vi "Main menu_4.vi"() -> ()   [LabVIEW 2022 SP3]
uses:
  <vilib>/event_ctls.llb/lveventtype.ctl
  <vilib>/Utility/file.llb/Write Delimited Spreadsheet (DBL).vi
panel:
  out "Close":bool
  in  "Close app":bool
  in  "?":T1(tab)
  in  "New plot":bool
  in  "Multicolumn Listbox":i32(listbox)
  in  "Close All plots":bool
  in  "CSV":bool
  in  "Start record":bool
  in  "Refresh \ntime (ms)":i32
  in  "Global Mode":enum32{"Item 0", "Item 1"}(radio)
  in  "Size bytes X #Traces":i32
  in  "Trace names":string(combo)
  in  "CTRL enable":bool
  in  "Save CTRL parameters":bool
  out "Total\ncontrols":i32
  in  "# Control":string(combo)
  in  "CS enable":bool
  out "Current CS status":i32
  in  "CS_IF_Params":T2 {"CS_Duty" min=0 max=1}
  out "Connected":bool
  out "Saved":bool
  in  "Save conf":bool
  in  "Port":i32
  in  "hostname":string
  in  "timeout ms":i32
  in  "Send message":bool
  in  "Process 2":i32
  in  "msj":string
  # "ctrl_if:0\nctrl: 2\nset parm: 2"
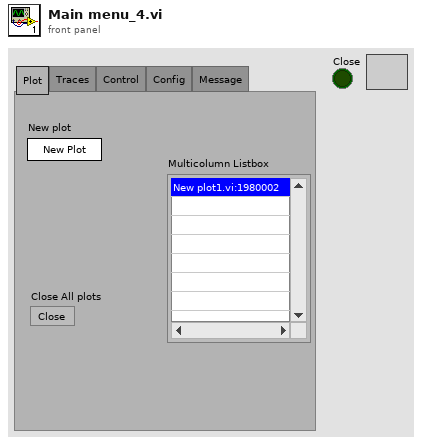
[diagram p1: front panel]
types:
  T1 = enum32{"Plot", "Traces", "Control", "Config", "Message"}
  T2 = cluster{"SET_PARAMETERS":i32, "CTLR":i32, "CS_Duty":sgl, "CTRL_IF_SET":i32}
  T3 = cluster{"Port":i32, "hostname":string, "status":bool, "timeout ms":i32, "TRACES_NAMES":string[], "Refresh time ms":i32, "Mode":enum32{"Item 0", "Item 1"}, "Start":bool, "DATA":sgl[][], "SIGNALS_NAMES":string[], "NB_SIGNALS":i32, "NB_TRACES":i32, "ID_TRACE":i32, "Mark":bool, "Counter":i32, "CTRLs_NAMES":string[], "NB_Ctrls":i32, "CS enable?":bool, "CS ID":i32}
  T4 = enum8{"Enabled", "Disabled", "Disabled and Grayed Out"}
  T5 = cluster{"TRACE_SIZE":i32, "CS_ID":i32, "TRACE ID":i32, "CMD":i32, "DATA PARAM":string}
  T6 = cluster{"TRACE_SIZE":i32, "CS_ID":i32, "TRACE ID":i32, "CMD":i32, "DATA(M)":i32}
  T7 = cluster{"timeout ms":i32, "remote port":u16, "Address":string}
  T8 = typedef "lveventtype.ctl" = enum32{"Null", "Timeout", "Annotation Menu Selection", "Annotation Menu Selection?", "App Instance Close", "App Instance Close?", "Autoscale Range Change", "Bookmark Info Change", "Cell Edit", "Cell Edit?", "Cursor Grab", "Cursor Grab?", "Cursor Menu Selection", "Cursor Menu Selection?", "Cursor Move", "Cursor Release", "Data Change", "Direction Change", "Display State Change", "Drag Ended", "Drag Enter", "Drag Leave", "Drag Over", "Drag Source Update", "Drag Starting", "Drag Starting?", "Drop", "Exec State Change", "Key Down", "Key Down?", "Key Repeat", "Key Repeat?", "Key Up", "Listbox Double Click", "Menu Activation?", "Menu Selection (App)", "Menu Selection? (App)", "Menu Selection (User)", "Mouse Down", "Mouse Down?", "Mouse Enter", "Mouse Leave", "Mouse Move", "Mouse Up", "Mouse Wheel", "NI Security User Change (App)", "Pane Size", "Panel Close", "Panel Close?", "Panel Resize", "Plot Attribute Change", "Scale Range Change", "Shortcut Menu Activation?", "Shortcut Menu Selection (App)", "Shortcut Menu Selection? (App)", "Shortcut Menu Selection (User)", "Tree Double Click", "Tree Drag", "Tree Drag?", "Tree Drop", "Tree Drop?", "Tree Item Close", "Tree Item Close?", "Tree Item Open", "Tree Item Open?", "User Event", "Value Change"}
  T9 = enum16{"open", "replace", "create", "open or create", "replace or create", "replace or create with confirmation"}
  T10 = enum16{"big-endian, network order", "native, host order", "little-endian"}
  T11 = cluster{"SIZE":i32, " TRACE DATA":sgl[], "TRACE_SIZE":i32, "NB_TRACES":i32, "NB_TRACED_SIGNALS":i32, "NAMES TRACED SIGNALS":string[], "NAMES TRACES":string[], "CS STATUS":i32, "NB_CSs":i32, "NAMES CSs":string[], "DATA (M)":sgl[], "CMD":i32}
  T12 = enum32{"invalid app kind", "Development System", "Run Time System", "Student Edition", "Embedded LabVIEW", "Evaluation", "Custom"}
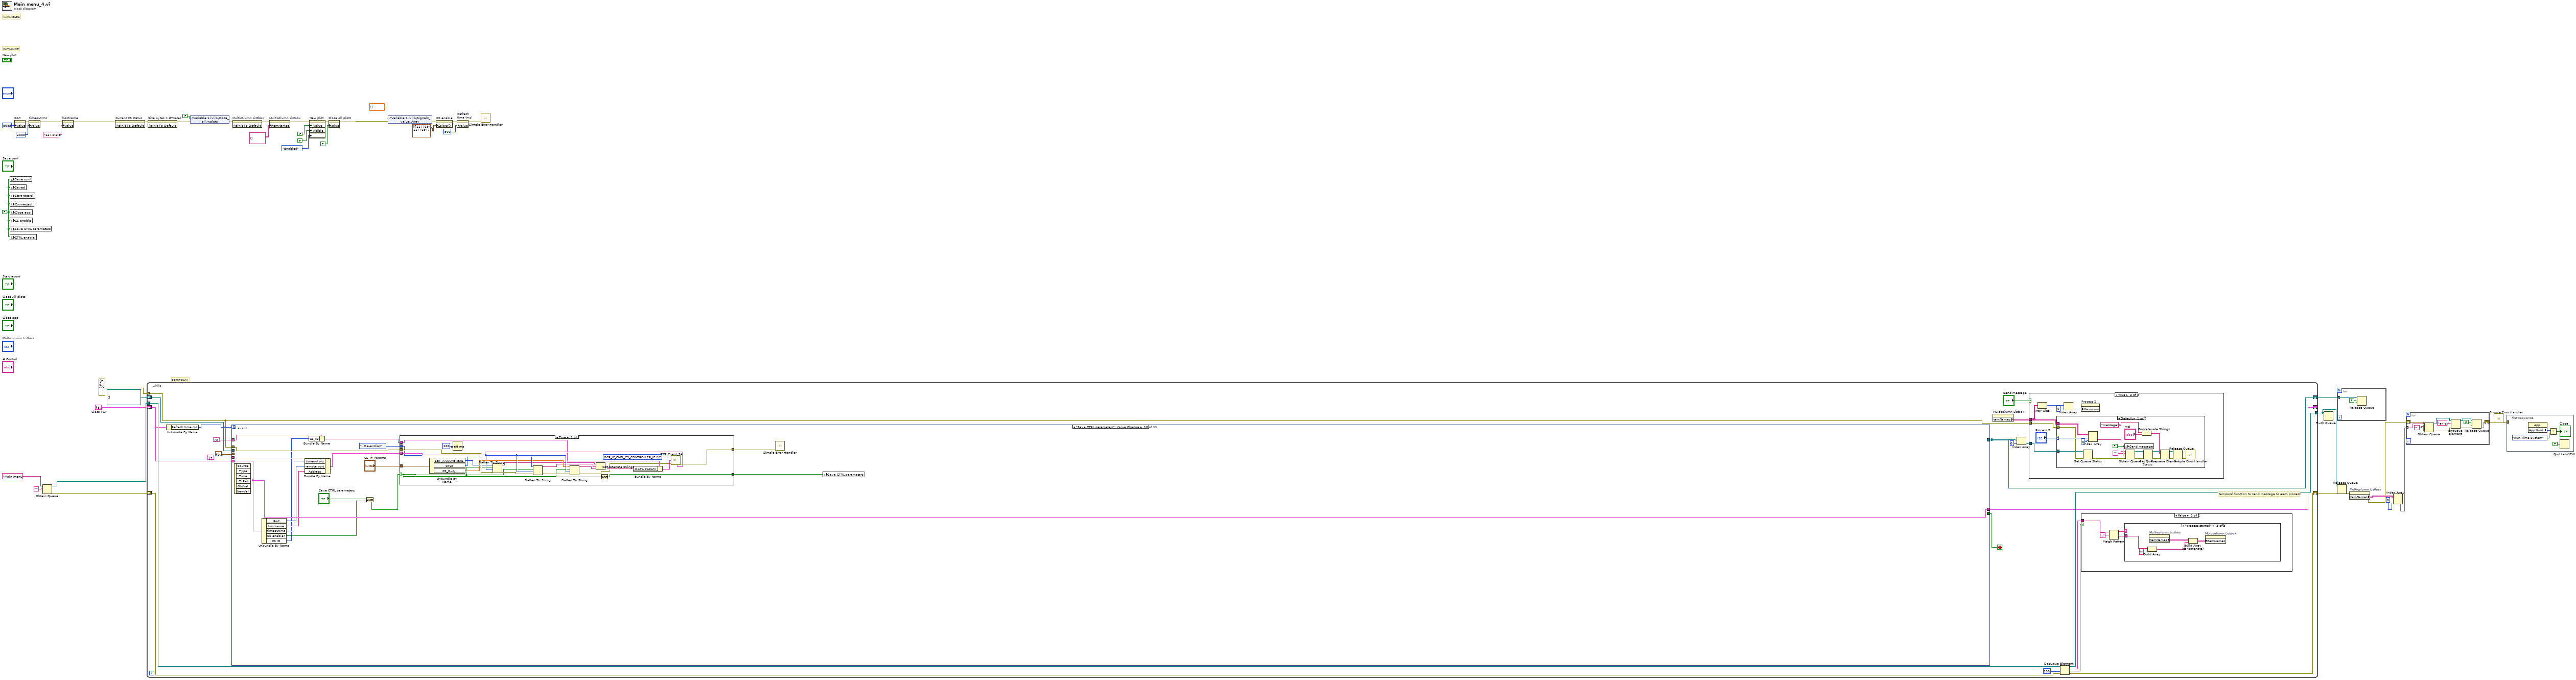
[diagram p0: block diagram]
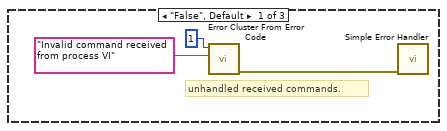
[diagram p4: hidden frame]
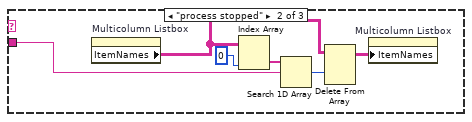
[diagram p5: hidden frame]
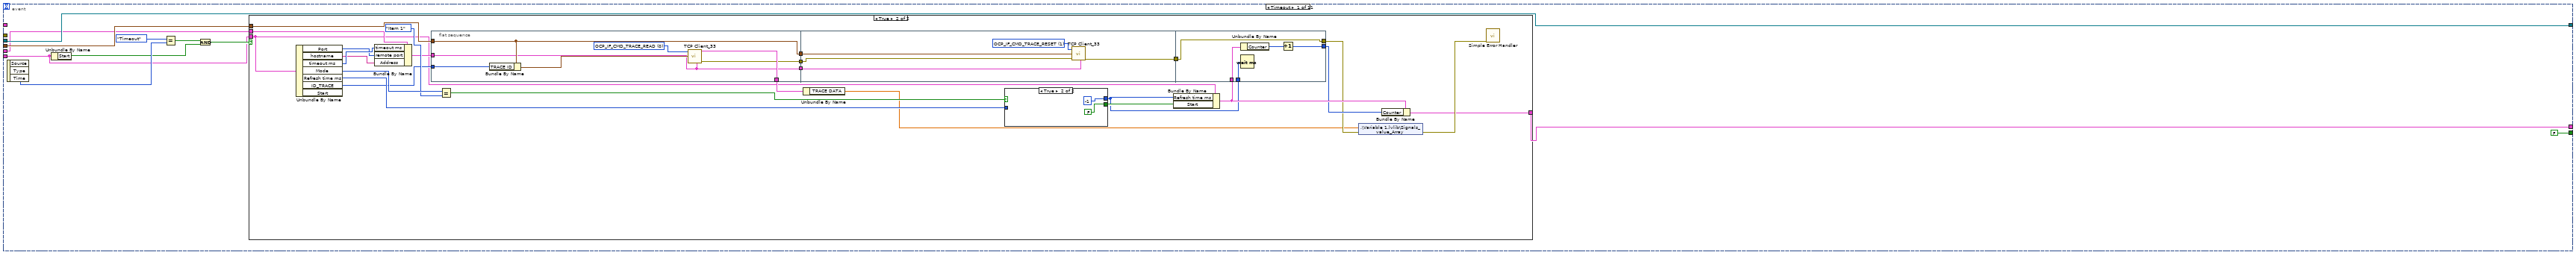
[diagram p7: hidden frame]
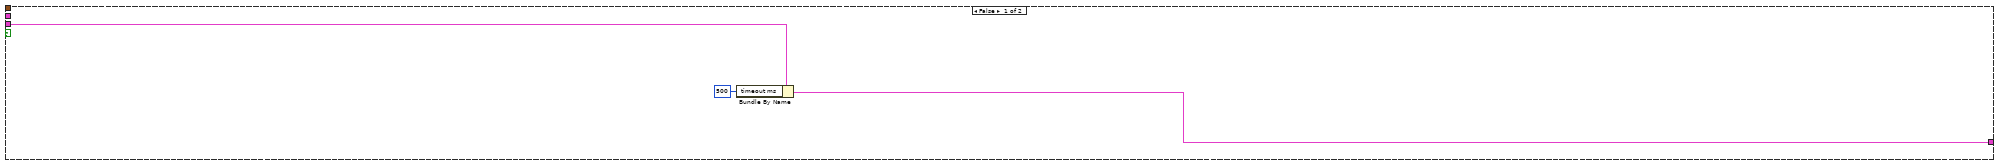
[diagram p8: hidden frame]
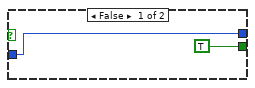
[diagram p9: hidden frame]
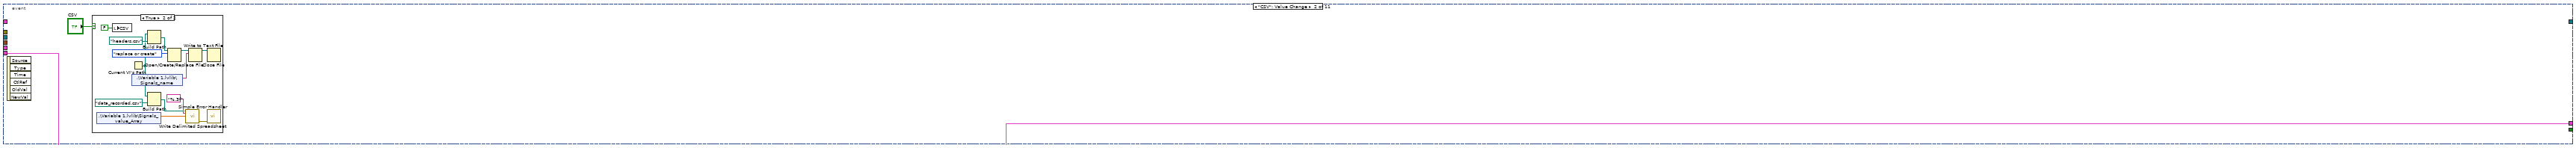
[diagram p10: hidden frame]
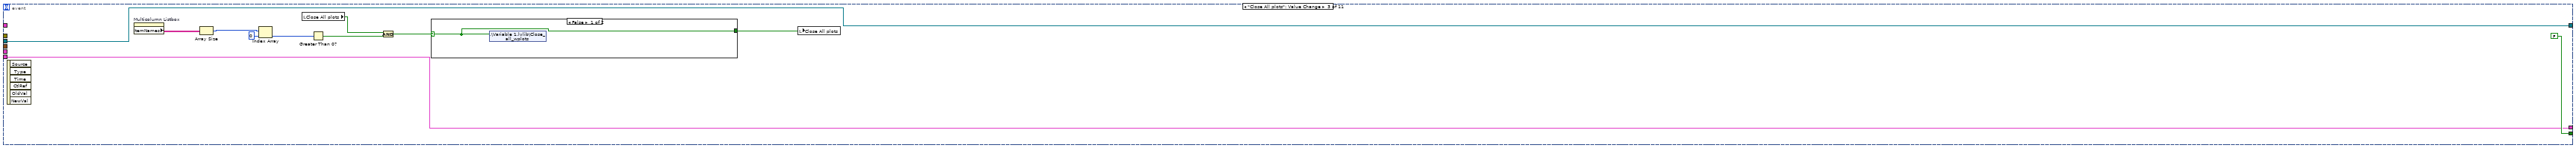
[diagram p12: hidden frame]
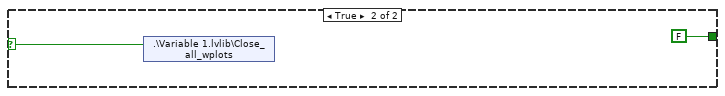
[diagram p13: hidden frame]
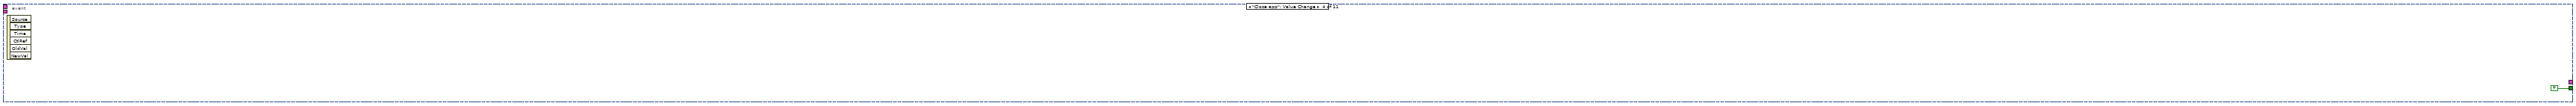
[diagram p14: hidden frame]
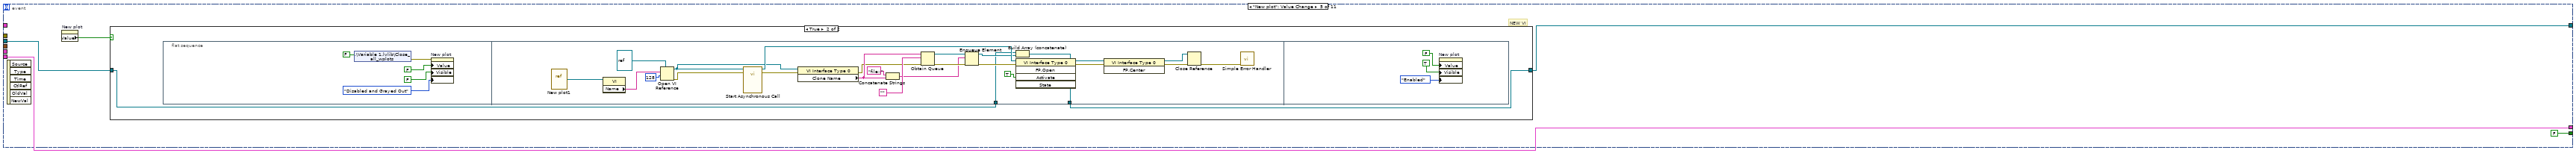
[diagram p15: hidden frame]
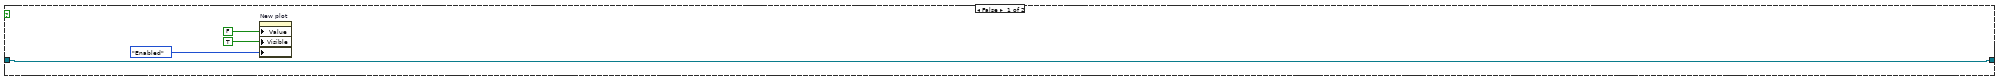
[diagram p16: hidden frame]
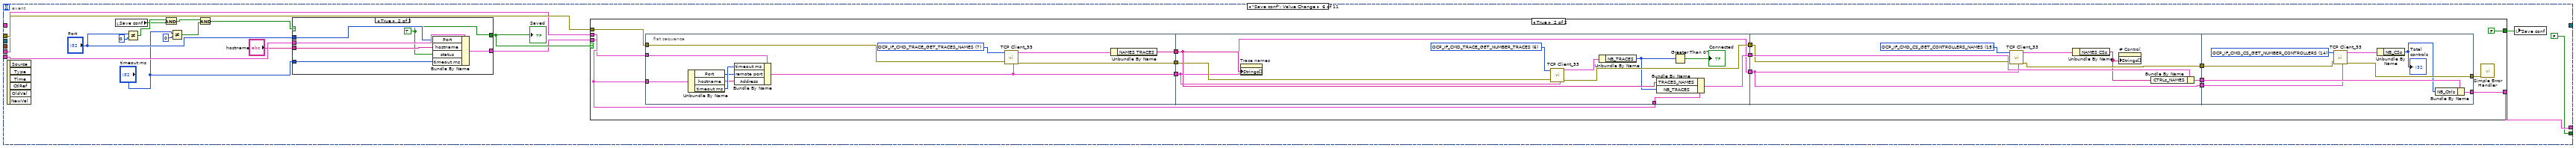
[diagram p17: hidden frame]
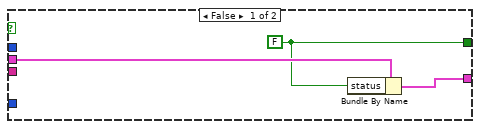
[diagram p19: hidden frame]
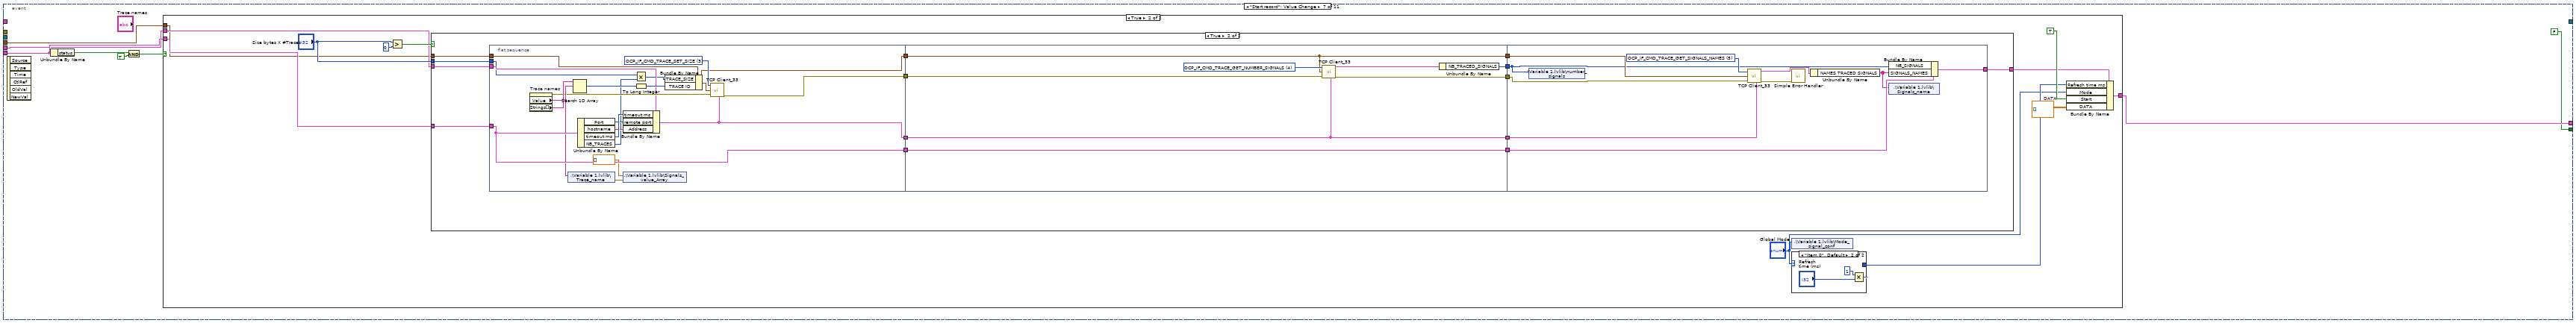
[diagram p20: hidden frame]
diagram:
  w22 = T3 {"Port"=8085, "hostname"="", "status"=FALSE, "timeout ms"=1000, "TRACES_NAMES"=[], "Refresh time ms"=500, "Mode"=enum."Item 0", "Start"=FALSE, "DATA"=[], "SIGNALS_NAMES"=[], "NB_SIGNALS"=0, "NB_TRACES"=0, "ID_TRACE"=0, "Mark"=FALSE, "Counter"=0, "CTRLs_NAMES"=[], "NB_Ctrls"=0, "CS enable?"=FALSE, "CS ID"=0}  # Class TCP
  w9 = FALSE ("Save conf")
  # "PROGRAM"
  # "INITIALIZE"
  # "VARIABLES"
  n1 = local write "Save conf"(w9) -> ()
  n2 = local write "Saved"(w9) -> ()
  n3 = local write "Start record"(w9) -> ()
  n4 = local write "Connected"(w9) -> ()
  n5 = local write "Close app"(w9) -> ()
  n6 = local write "CS enable"(w9) -> ()
  n7 = local write "Save CTRL parameters"(w9) -> ()
  n8 = local write "CTRL enable"(w9) -> ()
  n9 = property on="Port" class="DigNum (strict)"("Value"=8085) -> (error out=w20:errorcluster)  [unwired: 2 in, 1 out]
  n10 = property on="timeout ms" class="DigNum (strict)"(error in=w20, "Value"=2000 ("timeout ms")) -> (error out=w16:errorcluster)  [unwired: 1 in, 1 out]
  n11 = Obtain Queue(name (unnamed)="Main menu", element data type="") -> (queue out=w36:refnum<queue>, error out=w34:errorcluster)  [unwired: 3 in, 1 out]
  n12 = property on="hostname" class="Str"(error in=w16, "Value"="127.0.0.1" ("hostname")) -> (error out=w3:errorcluster)  [unwired: 1 in, 1 out]
  n13 = invoke on="Current CS status" class="DigNum (strict)" method="Reinit To Default"(error in=w3) -> (error out=w14:errorcluster)  [unwired: 2 in, 2 out]
  n14 = while {
    shift-right: [w48] -> w40
    shift-left: refnum<queue>[] [] -> [w63]
    tunnel: w36 -> [w62]
    tunnel: [w59] -> w26
    shift-right: [w53] -> w35
    shift-left: w34 -> [w58]
    shift-right: [w56] -> _
    shift-left: w22 -> [w55]
    tunnel: errorcluster {"status"=FALSE, "code"=0, "source"=""} ("error out") -> [w50]
    stop <- w64 stop-if-true
    # "temporal function to send message to each process"
    n15 = Unbundle By Name(w55) -> ("Refresh time ms"=w54:i32)
    n16 = event shown="[9] \"Save CTRL parameters\": Value Change" {
      selector: _ -> [_ _ _ _ _ _ _ _ _ _ _]
      dyn-events: _ -> [_ _ _ _ _ _ _ _ _ _ _]
      timeout: w54 -> [_ _ _ _ _ _ _ _ _ _ _]
      tunnel: [FALSE ("f") _ FALSE ("f") TRUE ("f") FALSE ("f") FALSE ("f") FALSE ("f") FALSE ("f") _ _ _] -> w64
      tunnel: [w119 _ w194 _ w202 _ _ _ _ _ _] -> w48
      tunnel: w63 -> [w119 _ w194 _ w201 _ _ _ _ _ _]
      tunnel: [w112 w169 w184 _ w199 w250 w328 w402 w445 w510 w561] -> w56
      tunnel: w55 -> [w113 w169 w184 _ w199 w258 w329 w402 w444 w510 w561]
      tunnel: w50 -> [_ _ _ _ _ w253 _ _ _ w511 w562]
      tunnel: T7 {"timeout ms"=2000, "remote port"=8085, "Address"="127.0.0.1"} ("Comunication Cluster") -> [w109 _ _ _ _ w243 w325 w406 w454 w507 w560]
      tunnel: T6 {"TRACE_SIZE"=0, "CS_ID"=0, "TRACE ID"=0, "CMD"=0, "DATA(M)"=0} ("Input Cluster") -> [w110 _ _ _ _ _ w324 w403 w453 _ _]
      tunnel: T5 {"TRACE_SIZE"=0, "CS_ID"=0, "TRACE ID"=0, "CMD"=0, "DATA PARAM"=""} ("Input Cluster") -> [_ _ _ _ _ _ _ _ _ w502 w555]
      event Timeout {
        n17 = event-data() -> ("Type"=w117:T8)  [unwired: 1 in, 2 out]
        n18 = Unbundle By Name(w113) -> ("Start"=w115:bool)
        n19 = Equal?(x=lveventtype."Timeout" ("Type"), y=w117) -> (x = y?=w116:bool)
        n20 = And(x=w116, y=w115) -> (x .and. y?=w114:bool)
        n21 = case shown="True" w114 {
          tunnel: w113 -> [w122 w123]
          tunnel: [w121 w137] -> w112
          tunnel: w110 -> [_ w126]
          tunnel: w109 -> [_ w125]
          frame False {
            n22 = Bundle By Name(cluster=w122, "timeout ms"=500) -> (w121:T3)
          }
          frame True {
            n23 = Unbundle By Name(w123) -> ("Port"=w131:i32, "hostname"=w130:string, "timeout ms"=w132:i32, "Mode"=w147:enum32{"Item 0", "Item 1"}, "Refresh time ms"=w144:i32, "ID_TRACE"=w141:i32)  [unwired: 1 out]
            n24 = Bundle By Name(cluster=w125, "timeout ms"=w132, "remote port"=w131, "Address"=w130) -> (w129:T7)
            n25 = flat-sequence {
              tunnel: w141 -> [w150]
              tunnel: [w154] -> w140
              tunnel: [w153] -> w139
              tunnel: w126 -> [w149]
              tunnel: [w149] -> w134
              tunnel: [w148] -> w133
              tunnel: w129 -> [w148]
              tunnel: w139 -> [w159]
              tunnel: w134 -> [w158]
              tunnel: w133 -> [w157]
              tunnel: [w155] -> w128
              tunnel: w138 -> [w164]
              tunnel: [w162] -> w136
              tunnel: w135 -> [w161]
              tunnel: w128 -> [w160]
              tunnel: [w160] -> w127
              frame #0 {
                w152 = 0 items=["OCP_IF_CMD_TRACE_READ", "OCP_IF_CMD_TRACE_RESET", "OCP_IF_CMD_TRACE_GET_SIZE", "OCP_IF_CMD_TRACE_SET_SIZE", "OCP_IF_CMD_TRACE_GET_NUMBER_SIGNALS", "OCP_IF_CMD_TRACE_GET_SIGNALS_NAMES", "OCP_IF_CMD_TRACE_GET_NUMBER_TRACES", "OCP_IF_CMD_TRACE_GET_TRACES_NAMES", "OCP_IF_CMD_TRACE_GET_ADDRESS", "OCP_IF_CMD_CS_STATUS", "OCP_IF_CMD_CS_ENABLE", "OCP_IF_CMD_CS_DISABLE", "OCP_IF_CMD_CS_CONTROLLER_IF", "OCP_IF_CMD_CS_HARDWARE_IF", "OCP_IF_CMD_CS_GET_NUMBER_CONTROLLERS", "OCP_IF_CMD_CS_GET_CONTROLLERS_NAMES", "OCP_IF_CMD_PLATFORM_ID", "OCP_IF_CMD_PLATFORM_IF", "OCP_IF_CMD_OPIL_UPDATE_MEASUREMENTS", "OCP_IF_CMD_OPIL_UPDATE_SIM_DATA", "OCP_IF_CMD_OPIL_RUN_CONTROL", "OCP_IF_CMD_OPIL_INITIALIZE_CONTROL", "OCP_IF_CMD_OPIL_GET_CONTROL", "OCP_IF_CMD_OPIL_GET_CONTROLLER_DATA", "OCP_IF_CMD_END"] ("CMD")
                n26 = Bundle By Name(cluster=w149, "TRACE ID"=w150) -> (w151:T6)
                n27 = call "TCP Client_33.vi"("CMD"=w152, "Input Cluster"=w151, "Comunication Cluster"=w148) -> ("Output cluster"=w154:T11, "error out"=w153:errorcluster)  [unwired: 5 in, 1 out]
              }
              frame #1 {
                w156 = 1 items=["OCP_IF_CMD_TRACE_READ", "OCP_IF_CMD_TRACE_RESET", "OCP_IF_CMD_TRACE_GET_SIZE", "OCP_IF_CMD_TRACE_SET_SIZE", "OCP_IF_CMD_TRACE_GET_NUMBER_SIGNALS", "OCP_IF_CMD_TRACE_GET_SIGNALS_NAMES", "OCP_IF_CMD_TRACE_GET_NUMBER_TRACES", "OCP_IF_CMD_TRACE_GET_TRACES_NAMES", "OCP_IF_CMD_TRACE_GET_ADDRESS", "OCP_IF_CMD_CS_STATUS", "OCP_IF_CMD_CS_ENABLE", "OCP_IF_CMD_CS_DISABLE", "OCP_IF_CMD_CS_CONTROLLER_IF", "OCP_IF_CMD_CS_HARDWARE_IF", "OCP_IF_CMD_CS_GET_NUMBER_CONTROLLERS", "OCP_IF_CMD_CS_GET_CONTROLLERS_NAMES", "OCP_IF_CMD_PLATFORM_ID", "OCP_IF_CMD_PLATFORM_IF", "OCP_IF_CMD_OPIL_UPDATE_MEASUREMENTS", "OCP_IF_CMD_OPIL_UPDATE_SIM_DATA", "OCP_IF_CMD_OPIL_RUN_CONTROL", "OCP_IF_CMD_OPIL_INITIALIZE_CONTROL", "OCP_IF_CMD_OPIL_GET_CONTROL", "OCP_IF_CMD_OPIL_GET_CONTROLLER_DATA", "OCP_IF_CMD_END"] ("CMD")
                n28 = call "TCP Client_33.vi"("CMD"=w156, "Input Cluster"=w158, "error in (no error)"=w159, "Comunication Cluster"=w157) -> ("error out"=w155:errorcluster)  [unwired: 4 in, 2 out]
              }
              frame #2 {
                n29 = Unbundle By Name(w164) -> ("Counter"=w163:i32)
                n30 = Wait (ms)(milliseconds to wait=w161) -> ()  [unwired: 1 out]
                n31 = Increment(x=w163) -> (x+1=w162:i32)
              }
            }
            n32 = Equal?(x=w147, y=enum32{"Item 0", "Item 1"}."Item 1" ("Mode")) -> (x = y?=w145:bool)
            n33 = Unbundle By Name(w140) -> ("TRACE DATA"=w124:sgl[])
            n34 = case shown="True" w145 {
              tunnel: [TRUE FALSE] -> w143
              tunnel: [w165 i8 -1 ("t")] -> w135
              tunnel: w144 -> [w165 _]
              frame False {
              }
              frame True {
              }
            }
            n35 = Bundle By Name(cluster=w123, "Refresh time ms"=w135, "Start"=w143) -> (w138:T3)
            n36 = shared-variable ".\\Variable 1.lvlib\\Signals_value_Array"(w124, error in=w127) -> (error out=w142:errorcluster)
            n37 = Bundle By Name(cluster=w138, "Counter"=w136) -> (w137:T3)
            n38 = call <vilib>:"Simple Error Handler.vi"("error in (no error)"=w142) -> ()  [unwired: 4 in, 5 out]
          }
        }
      }
      event "CSV": Value Change {
        n39 = event-data() -> ()  [unwired: 1 in, 6 out]
        n40 = case shown="True" "CSV" {
          frame False {
          }
          frame True {
            n41 = shared-variable ".\\Variable 1.lvlib\\Signals_value_Array"() -> (w180:dbl[])  [unwired: 1 in, 1 out]
            n42 = local write "CSV"(FALSE ("CSV")) -> ()
            n43 = Current VI's Path() -> (path=w171:path)
            n44 = shared-variable ".\\Variable 1.lvlib\\Signals_name"() -> (w174:string[])  [unwired: 1 in, 1 out]
            n45 = Build Path(base path=w171, name or relative path=path "headers.csv") -> (appended path=w177:path)
            n46 = Build Path(base path=w171, name or relative path=path "data_recorded.csv") -> (appended path=w179:path)
            n47 = Open/Create/Replace File(file path (use dialog)=w177, operation (0:open)=T9."replace or create") -> (refnum out=w175:refnum<file>)  [unwired: 4 in, 2 out]
            n48 = call-poly <vilib>:"Write Delimited Spreadsheet.vi"("file path (dialog if empty)"=w179, "format (%.3f)"="%.3f", "1D data"=w180) -> ("error out"=w181:errorcluster)  [unwired: 11 in, 1 out]
            n49 = Write to Text File(file (use dialog)=w175, text=w174) -> (refnum out=w173:refnum<file>)  [unwired: 2 in, 2 out]
            n50 = Close File(refnum=w173) -> ()  [unwired: 1 in, 2 out]
            n51 = call <vilib>:"Simple Error Handler.vi"("error in (no error)"=w181) -> ()  [unwired: 4 in, 5 out]
          }
        }
      }
      event "Close All plots": Value Change {
        n52 = event-data() -> ()  [unwired: 1 in, 6 out]
        n53 = property on="Multicolumn Listbox" class="MCListbox (strict)"() -> ("ItemNames"=w188:string[][])  [unwired: 2 in, 2 out]
        n54 = Array Size(array=w188) -> (size(s)=w192:i32[])
        n55 = Index Array(array=w192, index=0) -> (element=w190:i32)
        n56 = local read "Close All plots"() -> (w187:bool)
        n57 = Greater Than 0?(x=w190) -> (x > 0?=w185:bool)
        n58 = And(x=w187, y=w185) -> (x .and. y?=w186:bool)
        n59 = case shown="False" w186 {
          selector: w186 -> [w195 w196]
          tunnel: [w195 FALSE] -> w189
          frame False {
            n60 = shared-variable ".\\Variable 1.lvlib\\Close_all_wplots"(w195) -> ()  [unwired: 1 in, 1 out]
          }
          frame True {
            n61 = shared-variable ".\\Variable 1.lvlib\\Close_all_wplots"(w196) -> ()  [unwired: 1 in, 1 out]
          }
        }
        n62 = local write "Close All plots"(w189) -> ()
      }
      event "Close app": Value Change {
        n63 = event-data() -> ()  [unwired: 1 in, 6 out]
      }
      event "New plot": Value Change {
        # "NEW VI"
        n64 = event-data() -> ()  [unwired: 1 in, 6 out]
        n65 = property on="New plot" class="Bool (strict)"() -> ("Value"=w203:bool)  [unwired: 2 in, 2 out]
        n66 = case shown="True" w203 {
          tunnel: [w204 w209] -> w202
          tunnel: w201 -> [w204 w208]
          frame False {
            n67 = property on="New plot" class="Bool (strict)"("Value"=FALSE ("New plot"), "Visible"=TRUE, "DisabledEnum"=T4."Enabled" ("Disabled")) -> ()  [unwired: 2 in, 2 out]
          }
          frame True {
            n68 = flat-sequence {
              tunnel: [w220] -> w209
              tunnel: w208 -> [w219]
              frame #0 {
                n69 = shared-variable ".\\Variable 1.lvlib\\Close_all_wplots"(FALSE ("Close_all_wplots")) -> (error out=w210:errorcluster)  [unwired: 1 in]
                n70 = property on="New plot" class="Bool (strict)"(error in=w210, "Value"=FALSE ("New plot"), "Visible"=FALSE, "DisabledEnum"=T4."Disabled and Grayed Out" ("Disabled")) -> ()  [unwired: 1 in, 2 out]
              }
              frame #1 {
                n71 = vi-ref "New plot1.vi"() -> (w233:refnum<vi>)
                n72 = property class="VI"(reference=w233) -> ("Name"=w239:string)  [unwired: 1 in, 2 out]
                n73 = Open VI Reference(type specifier VI Refnum (for type only)=refnum<vi> refnum, vi path=w239, options=128) -> (vi reference=w230:refnum<vi>, error out=w235:errorcluster)  [unwired: 3 in]
                n74 = call-by-ref "Start Asynchronous Call"(reference=w230, error in=w235) -> (reference out=w234:refnum<vi>, error out=w224:errorcluster)  [unwired: 1 in, 1 out]
                n75 = property class="VI Interface Type 0"(reference=w230, error in=w224) -> (error out=w225:errorcluster, "Clone Name"=w227:string)  [unwired: 1 out]
                n76 = Concatenate Strings("file::" ("string"), w227) -> (w218:string)
                n77 = Obtain Queue(name (unnamed)=w227, element data type="", error in (no error)=w225) -> (queue out=w226:refnum<queue>, error out=w223:errorcluster)  [unwired: 2 in, 1 out]
                n78 = Enqueue Element(queue=w226, element=w218, error in (no error)=w223) -> (queue out=w221:refnum<queue>, error out=w222:errorcluster)  [unwired: 1 in, 1 out]
                n79 = Build Array (concatenate)(w219, w221) -> (w220:refnum<queue>[])
                n80 = invoke class="VI Interface Type 0" method="FP.Open"(reference=w234, error in=w222, "Activate"=TRUE ("Activate?")) -> (reference out=w232:refnum<vi>, error out=w217:errorcluster)  [unwired: 2 in, 3 out]
                n81 = invoke class="VI Interface Type 0" method="FP.Center"(reference=w232, error in=w217) -> (reference out=w231:refnum<vi>, error out=w216:errorcluster)  [unwired: 1 in, 1 out]
                n82 = Close Reference(reference=w231, error in (no error)=w216) -> (error out=w215:errorcluster)
                n83 = call <vilib>:"Simple Error Handler.vi"("error in (no error)"=w215) -> ()  [unwired: 4 in, 5 out]
              }
              frame #2 {
                n84 = property on="New plot" class="Bool (strict)"("Value"=FALSE ("Value (Signaling)"), "Visible"=TRUE, "DisabledEnum"=T4."Enabled" ("Disabled")) -> ()  [unwired: 2 in, 2 out]
              }
            }
          }
        }
      }
      event "Save conf": Value Change {
        n85 = event-data() -> ()  [unwired: 1 in, 6 out]
        n86 = local read "Save conf"() -> (w255:bool)
        n87 = Not Equal?(x="Port", y=0) -> (x != y?=w259:bool)
        n88 = And(x=w259, y=w255) -> (x .and. y?=w245:bool)
        n89 = Not Equal?(x="timeout ms", y=0) -> (x != y?=w247:bool)
        n90 = And(x=w245, y=w247) -> (x .and. y?=w246:bool)
        n91 = case shown="True" w246 {
          tunnel: [w315 w320] -> w254
          tunnel: "Port" -> [_ w322]
          tunnel: "hostname" -> [_ w321]
          tunnel: [w317 w318] -> w251
          tunnel: w258 -> [w316 w323]
          tunnel: "timeout ms" -> [_ w319]
          frame False {
            w315 = FALSE
            n92 = Bundle By Name(cluster=w316, "status"=w315) -> (w317:T3)
          }
          frame True {
            w320 = TRUE
            n93 = Bundle By Name(cluster=w323, "Port"=w322, "hostname"=w321, "status"=w320, "timeout ms"=w319) -> (w318:T3)
          }
        }
        "Saved" <- w254
        n94 = case shown="True" w254 {
          selector: w254 -> [w261 _]
          tunnel: w253 -> [_ w265]
          tunnel: [w261 FALSE] -> w252
          tunnel: w251 -> [w262 w276]
          tunnel: [w262 w275] -> w250
          tunnel: w243 -> [_ w263]
          frame False {
          }
          frame True {
            n95 = flat-sequence {
              tunnel: w276 -> [w288]
              tunnel: [w282] -> w274
              tunnel: [w281] -> w273
              tunnel: [w280] -> w272
              tunnel: w265 -> [w279]
              tunnel: w263 -> [w278]
              tunnel: w276 -> [w298]
              tunnel: w274 -> [w296]
              tunnel: w273 -> [w295]
              tunnel: w272 -> [w291]
              tunnel: [w297] -> w271
              tunnel: [w292] -> w269
              tunnel: [w291] -> w268
              tunnel: w271 -> [w306]
              tunnel: [w300] -> w270
              tunnel: w269 -> [w305]
              tunnel: w268 -> [w302]
              tunnel: [w303] -> w267
              tunnel: [w302] -> w266
              tunnel: [w310] -> w275
              tunnel: w270 -> [w314]
              tunnel: w267 -> [w313]
              tunnel: w266 -> [w312]
              tunnel: [w308] -> w264
              frame #0 {
                w287 = 7 items=["OCP_IF_CMD_TRACE_READ", "OCP_IF_CMD_TRACE_RESET", "OCP_IF_CMD_TRACE_GET_SIZE", "OCP_IF_CMD_TRACE_SET_SIZE", "OCP_IF_CMD_TRACE_GET_NUMBER_SIGNALS", "OCP_IF_CMD_TRACE_GET_SIGNALS_NAMES", "OCP_IF_CMD_TRACE_GET_NUMBER_TRACES", "OCP_IF_CMD_TRACE_GET_TRACES_NAMES", "OCP_IF_CMD_TRACE_GET_ADDRESS", "OCP_IF_CMD_CS_STATUS", "OCP_IF_CMD_CS_ENABLE", "OCP_IF_CMD_CS_DISABLE", "OCP_IF_CMD_CS_CONTROLLER_IF", "OCP_IF_CMD_CS_HARDWARE_IF", "OCP_IF_CMD_CS_GET_NUMBER_CONTROLLERS", "OCP_IF_CMD_CS_GET_CONTROLLERS_NAMES", "OCP_IF_CMD_PLATFORM_ID", "OCP_IF_CMD_PLATFORM_IF", "OCP_IF_CMD_OPIL_UPDATE_MEASUREMENTS", "OCP_IF_CMD_OPIL_UPDATE_SIM_DATA", "OCP_IF_CMD_OPIL_RUN_CONTROL", "OCP_IF_CMD_OPIL_INITIALIZE_CONTROL", "OCP_IF_CMD_OPIL_GET_CONTROL", "OCP_IF_CMD_OPIL_GET_CONTROLLER_DATA", "OCP_IF_CMD_END"] ("CMD")
                n96 = Unbundle By Name(w288) -> ("Port"=w284:i32, "hostname"=w283:string, "timeout ms"=w285:i32)
                n97 = Bundle By Name(cluster=w278, "timeout ms"=w285, "remote port"=w284, "Address"=w283) -> (w280:T7)
                n98 = call "TCP Client_33.vi"("CMD"=w287, "error in (no error)"=w279, "Comunication Cluster"=w280) -> ("Output cluster"=w286:T11, "error out"=w281:errorcluster)  [unwired: 5 in, 1 out]
                n99 = Unbundle By Name(w286) -> ("NAMES TRACES"=w282:string[])
              }
              frame #1 {
                w294 = 6 items=["OCP_IF_CMD_TRACE_READ", "OCP_IF_CMD_TRACE_RESET", "OCP_IF_CMD_TRACE_GET_SIZE", "OCP_IF_CMD_TRACE_SET_SIZE", "OCP_IF_CMD_TRACE_GET_NUMBER_SIGNALS", "OCP_IF_CMD_TRACE_GET_SIGNALS_NAMES", "OCP_IF_CMD_TRACE_GET_NUMBER_TRACES", "OCP_IF_CMD_TRACE_GET_TRACES_NAMES", "OCP_IF_CMD_TRACE_GET_ADDRESS", "OCP_IF_CMD_CS_STATUS", "OCP_IF_CMD_CS_ENABLE", "OCP_IF_CMD_CS_DISABLE", "OCP_IF_CMD_CS_CONTROLLER_IF", "OCP_IF_CMD_CS_HARDWARE_IF", "OCP_IF_CMD_CS_GET_NUMBER_CONTROLLERS", "OCP_IF_CMD_CS_GET_CONTROLLERS_NAMES", "OCP_IF_CMD_PLATFORM_ID", "OCP_IF_CMD_PLATFORM_IF", "OCP_IF_CMD_OPIL_UPDATE_MEASUREMENTS", "OCP_IF_CMD_OPIL_UPDATE_SIM_DATA", "OCP_IF_CMD_OPIL_RUN_CONTROL", "OCP_IF_CMD_OPIL_INITIALIZE_CONTROL", "OCP_IF_CMD_OPIL_GET_CONTROL", "OCP_IF_CMD_OPIL_GET_CONTROLLER_DATA", "OCP_IF_CMD_END"] ("CMD")
                n100 = property on="Trace names" class="CmbBox"("Strings[]"=w296) -> ()  [unwired: 2 in, 2 out]
                n101 = call "TCP Client_33.vi"("CMD"=w294, "error in (no error)"=w295, "Comunication Cluster"=w291) -> ("Output cluster"=w293:T11, "error out"=w292:errorcluster)  [unwired: 5 in, 1 out]
                n102 = Unbundle By Name(w293) -> ("NB_TRACES"=w290:i32)
                n103 = Bundle By Name(cluster=w298, "TRACES_NAMES"=w296, "NB_TRACES"=w290) -> (w297:T3)
                n104 = Greater Than 0?(x=w290) -> (x > 0?=→"Connected":bool)
              }
              frame #2 {
                w304 = 15 items=["OCP_IF_CMD_TRACE_READ", "OCP_IF_CMD_TRACE_RESET", "OCP_IF_CMD_TRACE_GET_SIZE", "OCP_IF_CMD_TRACE_SET_SIZE", "OCP_IF_CMD_TRACE_GET_NUMBER_SIGNALS", "OCP_IF_CMD_TRACE_GET_SIGNALS_NAMES", "OCP_IF_CMD_TRACE_GET_NUMBER_TRACES", "OCP_IF_CMD_TRACE_GET_TRACES_NAMES", "OCP_IF_CMD_TRACE_GET_ADDRESS", "OCP_IF_CMD_CS_STATUS", "OCP_IF_CMD_CS_ENABLE", "OCP_IF_CMD_CS_DISABLE", "OCP_IF_CMD_CS_CONTROLLER_IF", "OCP_IF_CMD_CS_HARDWARE_IF", "OCP_IF_CMD_CS_GET_NUMBER_CONTROLLERS", "OCP_IF_CMD_CS_GET_CONTROLLERS_NAMES", "OCP_IF_CMD_PLATFORM_ID", "OCP_IF_CMD_PLATFORM_IF", "OCP_IF_CMD_OPIL_UPDATE_MEASUREMENTS", "OCP_IF_CMD_OPIL_UPDATE_SIM_DATA", "OCP_IF_CMD_OPIL_RUN_CONTROL", "OCP_IF_CMD_OPIL_INITIALIZE_CONTROL", "OCP_IF_CMD_OPIL_GET_CONTROL", "OCP_IF_CMD_OPIL_GET_CONTROLLER_DATA", "OCP_IF_CMD_END"] ("CMD")
                n105 = call "TCP Client_33.vi"("CMD"=w304, "error in (no error)"=w305, "Comunication Cluster"=w302) -> ("Output cluster"=w301:T11, "error out"=w303:errorcluster)  [unwired: 5 in, 1 out]
                n106 = Unbundle By Name(w301) -> ("NAMES CSs"=w299:string[])
                n107 = property on="# Control" class="CmbBox"("Strings[]"=w299) -> ()  [unwired: 2 in, 2 out]
                n108 = Bundle By Name(cluster=w306, "CTRLs_NAMES"=w299) -> (w300:T3)
              }
              frame #3 {
                w311 = 14 items=["OCP_IF_CMD_TRACE_READ", "OCP_IF_CMD_TRACE_RESET", "OCP_IF_CMD_TRACE_GET_SIZE", "OCP_IF_CMD_TRACE_SET_SIZE", "OCP_IF_CMD_TRACE_GET_NUMBER_SIGNALS", "OCP_IF_CMD_TRACE_GET_SIGNALS_NAMES", "OCP_IF_CMD_TRACE_GET_NUMBER_TRACES", "OCP_IF_CMD_TRACE_GET_TRACES_NAMES", "OCP_IF_CMD_TRACE_GET_ADDRESS", "OCP_IF_CMD_CS_STATUS", "OCP_IF_CMD_CS_ENABLE", "OCP_IF_CMD_CS_DISABLE", "OCP_IF_CMD_CS_CONTROLLER_IF", "OCP_IF_CMD_CS_HARDWARE_IF", "OCP_IF_CMD_CS_GET_NUMBER_CONTROLLERS", "OCP_IF_CMD_CS_GET_CONTROLLERS_NAMES", "OCP_IF_CMD_PLATFORM_ID", "OCP_IF_CMD_PLATFORM_IF", "OCP_IF_CMD_OPIL_UPDATE_MEASUREMENTS", "OCP_IF_CMD_OPIL_UPDATE_SIM_DATA", "OCP_IF_CMD_OPIL_RUN_CONTROL", "OCP_IF_CMD_OPIL_INITIALIZE_CONTROL", "OCP_IF_CMD_OPIL_GET_CONTROL", "OCP_IF_CMD_OPIL_GET_CONTROLLER_DATA", "OCP_IF_CMD_END"] ("CMD")
                n109 = call "TCP Client_33.vi"("CMD"=w311, "error in (no error)"=w313, "Comunication Cluster"=w312) -> ("Output cluster"=w309:T11, "error out"=w308:errorcluster)  [unwired: 5 in, 1 out]
                n110 = Unbundle By Name(w309) -> ("NB_CSs"=w307:i32)
                "Total\ncontrols" <- w307
                n111 = Bundle By Name(cluster=w314, "NB_Ctrls"=w307) -> (w310:T3)
              }
            }
            n112 = call <vilib>:"Simple Error Handler.vi"("error in (no error)"=w264) -> ()  [unwired: 4 in, 5 out]
          }
        }
        n113 = local write "Save conf"(w252) -> ()
      }
      event "Start record": Value Change {
        n114 = event-data() -> ()  [unwired: 1 in, 6 out]
        n115 = Unbundle By Name(w329) -> ("status"=w331:bool)
        n116 = And(x=w331, y=TRUE) -> (x .and. y?=w330:bool)
        n117 = case shown="True" w330 {
          tunnel: w329 -> [w332 w338]
          tunnel: [w332 w344] -> w328
          tunnel: w325 -> [_ w335]
          tunnel: w324 -> [_ w334]
          frame False {
          }
          frame True {
            w333 = sgl[][] []  # DATA
            n118 = Greater?(x="Size bytes X #Traces", y=0) -> (0:w340:bool)
            n119 = case shown="True" w340 {
              tunnel: "Size bytes X #Traces" -> [_ w359]
              tunnel: w338 -> [w345 w358]
              tunnel: [w345 w354] -> w337
              tunnel: w335 -> [_ w347]
              tunnel: w334 -> [_ w346]
              frame False {
              }
              frame True {
                n120 = flat-sequence {
                  tunnel: w359 -> [w363]
                  tunnel: w358 -> [w379]
                  tunnel: [w375] -> w357
                  tunnel: [w379] -> w356
                  tunnel: [w368] -> w353
                  tunnel: [w367] -> w352
                  tunnel: w347 -> [w366]
                  tunnel: w346 -> [w365]
                  tunnel: w357 -> [w386]
                  tunnel: w356 -> [w387]
                  tunnel: [w387] -> w355
                  tunnel: w353 -> [w380]
                  tunnel: w352 -> [w381]
                  tunnel: [w383] -> w351
                  tunnel: [w382] -> w350
                  tunnel: [w381] -> w349
                  tunnel: [w380] -> w348
                  tunnel: w355 -> [w397]
                  tunnel: [w396] -> w354
                  tunnel: w351 -> [w388]
                  tunnel: w350 -> [w392]
                  tunnel: w349 -> [w390]
                  tunnel: w348 -> [w389]
                  frame #0 {
                    w374 = 3 items=["OCP_IF_CMD_TRACE_READ", "OCP_IF_CMD_TRACE_RESET", "OCP_IF_CMD_TRACE_GET_SIZE", "OCP_IF_CMD_TRACE_SET_SIZE", "OCP_IF_CMD_TRACE_GET_NUMBER_SIGNALS", "OCP_IF_CMD_TRACE_GET_SIGNALS_NAMES", "OCP_IF_CMD_TRACE_GET_NUMBER_TRACES", "OCP_IF_CMD_TRACE_GET_TRACES_NAMES", "OCP_IF_CMD_TRACE_GET_ADDRESS", "OCP_IF_CMD_CS_STATUS", "OCP_IF_CMD_CS_ENABLE", "OCP_IF_CMD_CS_DISABLE", "OCP_IF_CMD_CS_CONTROLLER_IF", "OCP_IF_CMD_CS_HARDWARE_IF", "OCP_IF_CMD_CS_GET_NUMBER_CONTROLLERS", "OCP_IF_CMD_CS_GET_CONTROLLERS_NAMES", "OCP_IF_CMD_PLATFORM_ID", "OCP_IF_CMD_PLATFORM_IF", "OCP_IF_CMD_OPIL_UPDATE_MEASUREMENTS", "OCP_IF_CMD_OPIL_UPDATE_SIM_DATA", "OCP_IF_CMD_OPIL_RUN_CONTROL", "OCP_IF_CMD_OPIL_INITIALIZE_CONTROL", "OCP_IF_CMD_OPIL_GET_CONTROL", "OCP_IF_CMD_OPIL_GET_CONTROLLER_DATA", "OCP_IF_CMD_END"] ("CMD")
                    n121 = property on="Trace names" class="CmbBox"() -> (error out=w370:errorcluster, "Value"=w376:string, "Strings[]"=w378:string[])  [unwired: 2 in, 1 out]
                    n122 = shared-variable ".\\Variable 1.lvlib\\Trace_name"(w376) -> (error out=w361:errorcluster)  [unwired: 1 in]
                    n123 = Search 1D Array(1D array=w378, element=w376) -> (index of element=w377:i32)  [unwired: 1 in]
                    n124 = Unbundle By Name(w379) -> ("Port"=w372:i32, "hostname"=w371:string, "timeout ms"=w373:i32, "NB_TRACES"=w364:i32)
                    n125 = Bundle By Name(cluster=w366, "timeout ms"=w373, "remote port"=w372, "Address"=w371) -> (w367:T7)
                    n126 = shared-variable ".\\Variable 1.lvlib\\Signals_value_Array"(dbl[] [] ("Signals_value_Array"), error in=w361) -> ()  [unwired: 1 out]
                    n127 = Multiply(x=w363, y=w364) -> (x*y=w362:i32)
                    n128 = To Long Integer(number=w377) -> (32bit integer=w369:i32)
                    n129 = Bundle By Name(cluster=w365, "TRACE_SIZE"=w362, "TRACE ID"=w369) -> (w368:T6)
                    n130 = call "TCP Client_33.vi"("CMD"=w374, "Input Cluster"=w368, "error in (no error)"=w370, "Comunication Cluster"=w367) -> ("error out"=w375:errorcluster)  [unwired: 4 in, 2 out]
                  }
                  frame #1 {
                    w385 = 4 items=["OCP_IF_CMD_TRACE_READ", "OCP_IF_CMD_TRACE_RESET", "OCP_IF_CMD_TRACE_GET_SIZE", "OCP_IF_CMD_TRACE_SET_SIZE", "OCP_IF_CMD_TRACE_GET_NUMBER_SIGNALS", "OCP_IF_CMD_TRACE_GET_SIGNALS_NAMES", "OCP_IF_CMD_TRACE_GET_NUMBER_TRACES", "OCP_IF_CMD_TRACE_GET_TRACES_NAMES", "OCP_IF_CMD_TRACE_GET_ADDRESS", "OCP_IF_CMD_CS_STATUS", "OCP_IF_CMD_CS_ENABLE", "OCP_IF_CMD_CS_DISABLE", "OCP_IF_CMD_CS_CONTROLLER_IF", "OCP_IF_CMD_CS_HARDWARE_IF", "OCP_IF_CMD_CS_GET_NUMBER_CONTROLLERS", "OCP_IF_CMD_CS_GET_CONTROLLERS_NAMES", "OCP_IF_CMD_PLATFORM_ID", "OCP_IF_CMD_PLATFORM_IF", "OCP_IF_CMD_OPIL_UPDATE_MEASUREMENTS", "OCP_IF_CMD_OPIL_UPDATE_SIM_DATA", "OCP_IF_CMD_OPIL_RUN_CONTROL", "OCP_IF_CMD_OPIL_INITIALIZE_CONTROL", "OCP_IF_CMD_OPIL_GET_CONTROL", "OCP_IF_CMD_OPIL_GET_CONTROLLER_DATA", "OCP_IF_CMD_END"] ("CMD")
                    n131 = call "TCP Client_33.vi"("CMD"=w385, "Input Cluster"=w380, "error in (no error)"=w386, "Comunication Cluster"=w381) -> ("Output cluster"=w384:T11, "error out"=w382:errorcluster)  [unwired: 4 in, 1 out]
                    n132 = Unbundle By Name(w384) -> ("NB_TRACED_SIGNALS"=w383:i32)
                  }
                  frame #2 {
                    w391 = 5 items=["OCP_IF_CMD_TRACE_READ", "OCP_IF_CMD_TRACE_RESET", "OCP_IF_CMD_TRACE_GET_SIZE", "OCP_IF_CMD_TRACE_SET_SIZE", "OCP_IF_CMD_TRACE_GET_NUMBER_SIGNALS", "OCP_IF_CMD_TRACE_GET_SIGNALS_NAMES", "OCP_IF_CMD_TRACE_GET_NUMBER_TRACES", "OCP_IF_CMD_TRACE_GET_TRACES_NAMES", "OCP_IF_CMD_TRACE_GET_ADDRESS", "OCP_IF_CMD_CS_STATUS", "OCP_IF_CMD_CS_ENABLE", "OCP_IF_CMD_CS_DISABLE", "OCP_IF_CMD_CS_CONTROLLER_IF", "OCP_IF_CMD_CS_HARDWARE_IF", "OCP_IF_CMD_CS_GET_NUMBER_CONTROLLERS", "OCP_IF_CMD_CS_GET_CONTROLLERS_NAMES", "OCP_IF_CMD_PLATFORM_ID", "OCP_IF_CMD_PLATFORM_IF", "OCP_IF_CMD_OPIL_UPDATE_MEASUREMENTS", "OCP_IF_CMD_OPIL_UPDATE_SIM_DATA", "OCP_IF_CMD_OPIL_RUN_CONTROL", "OCP_IF_CMD_OPIL_INITIALIZE_CONTROL", "OCP_IF_CMD_OPIL_GET_CONTROL", "OCP_IF_CMD_OPIL_GET_CONTROLLER_DATA", "OCP_IF_CMD_END"] ("CMD")
                    n133 = shared-variable ".\\Variable 1.lvlib\\number_signals"(w388) -> ()  [unwired: 1 in, 1 out]
                    n134 = call "TCP Client_33.vi"("CMD"=w391, "Input Cluster"=w389, "error in (no error)"=w392, "Comunication Cluster"=w390) -> ("Output cluster"=w395:T11, "error out"=w393:errorcluster)  [unwired: 4 in, 1 out]
                    n135 = call <vilib>:"Simple Error Handler.vi"("error in (no error)"=w393) -> ()  [unwired: 4 in, 5 out]
                    n136 = Unbundle By Name(w395) -> ("NAMES TRACED SIGNALS"=w394:string[])
                    n137 = Bundle By Name(cluster=w397, "NB_SIGNALS"=w388, "SIGNALS_NAMES"=w394) -> (w396:T3)
                    n138 = shared-variable ".\\Variable 1.lvlib\\Signals_name"(w394) -> ()  [unwired: 1 in, 1 out]
                  }
                }
              }
            }
            n139 = shared-variable ".\\Variable 1.lvlib\\Mode_signal_conf"("Global Mode") -> ()  [unwired: 1 in, 1 out]
            n140 = case shown="\"Item 0\", Default" "Global Mode" {
              tunnel: [200 ("Refresh time (sec)") w399] -> w342
              frame "Item 1" {
              }
              frame "Item 0", Default {
                n141 = Multiply(x=1, y="Refresh \ntime (ms)") -> (x*y=w399:i32)
              }
            }
            n142 = Bundle By Name(cluster=w337, "Refresh time ms"=w342, "Mode"="Global Mode", "Start"=TRUE, "DATA"=w333) -> (w344:T3)
          }
        }
      }
      event "Trace names", "# Control": Value Change {
        n143 = event-data() -> ()  [unwired: 1 in, 6 out]
        n144 = Unbundle By Name(w402) -> ("Port"=w410:i32, "hostname"=w409:string, "timeout ms"=w408:i32)
        n145 = Bundle By Name(cluster=w406, "timeout ms"=w408, "remote port"=w410, "Address"=w409) -> (w405:T7)
        n146 = flat-sequence {
          tunnel: w403 -> [w424]
          tunnel: [w424] -> w411
          tunnel: [w426] -> w407
          tunnel: w405 -> [w425]
          tunnel: [w425] -> w404
          tunnel: [w437] -> w412
          tunnel: w411 -> [w441]
          tunnel: w407 -> [w436]
          tunnel: w404 -> [w435]
          frame #0 {
            w427 = 2 items=["OCP_IF_CMD_TRACE_READ", "OCP_IF_CMD_TRACE_RESET", "OCP_IF_CMD_TRACE_GET_SIZE", "OCP_IF_CMD_TRACE_SET_SIZE", "OCP_IF_CMD_TRACE_GET_NUMBER_SIGNALS", "OCP_IF_CMD_TRACE_GET_SIGNALS_NAMES", "OCP_IF_CMD_TRACE_GET_NUMBER_TRACES", "OCP_IF_CMD_TRACE_GET_TRACES_NAMES", "OCP_IF_CMD_TRACE_GET_ADDRESS", "OCP_IF_CMD_CS_STATUS", "OCP_IF_CMD_CS_ENABLE", "OCP_IF_CMD_CS_DISABLE", "OCP_IF_CMD_CS_CONTROLLER_IF", "OCP_IF_CMD_CS_HARDWARE_IF", "OCP_IF_CMD_CS_GET_NUMBER_CONTROLLERS", "OCP_IF_CMD_CS_GET_CONTROLLERS_NAMES", "OCP_IF_CMD_PLATFORM_ID", "OCP_IF_CMD_PLATFORM_IF", "OCP_IF_CMD_OPIL_UPDATE_MEASUREMENTS", "OCP_IF_CMD_OPIL_UPDATE_SIM_DATA", "OCP_IF_CMD_OPIL_RUN_CONTROL", "OCP_IF_CMD_OPIL_INITIALIZE_CONTROL", "OCP_IF_CMD_OPIL_GET_CONTROL", "OCP_IF_CMD_OPIL_GET_CONTROLLER_DATA", "OCP_IF_CMD_END"] ("CMD")
            n147 = property on="Trace names" class="CmbBox"() -> ("Value"=w419:string, "Strings[]"=w420:string[])  [unwired: 2 in, 2 out]
            n148 = Search 1D Array(1D array=w420, element=w419) -> (index of element=w415:i32)  [unwired: 1 in]
            n149 = Less Than 0?(x=w415) -> (x < 0?=w416:bool)
            n150 = Select(t=0, s=w416, f=w415) -> (s? t:f=w414:i32)
            n151 = To Long Integer(number=w414) -> (32bit integer=w418:i32)
            n152 = Bundle By Name(cluster=w424, "TRACE ID"=w418) -> (w423:T6)
            n153 = call "TCP Client_33.vi"("CMD"=w427, "Input Cluster"=w423, "Comunication Cluster"=w425) -> ("Output cluster"=w421:T11, "error out"=w426:errorcluster)  [unwired: 5 in, 1 out]
            n154 = Unbundle By Name(w421) -> ("TRACE_SIZE"=w422:i32)
            n155 = property on="Size bytes X #Traces" class="DigNum (strict)"("Value"=w422) -> ()  [unwired: 2 in, 2 out]
          }
          frame #1 {
            w440 = 9 items=["OCP_IF_CMD_TRACE_READ", "OCP_IF_CMD_TRACE_RESET", "OCP_IF_CMD_TRACE_GET_SIZE", "OCP_IF_CMD_TRACE_SET_SIZE", "OCP_IF_CMD_TRACE_GET_NUMBER_SIGNALS", "OCP_IF_CMD_TRACE_GET_SIGNALS_NAMES", "OCP_IF_CMD_TRACE_GET_NUMBER_TRACES", "OCP_IF_CMD_TRACE_GET_TRACES_NAMES", "OCP_IF_CMD_TRACE_GET_ADDRESS", "OCP_IF_CMD_CS_STATUS", "OCP_IF_CMD_CS_ENABLE", "OCP_IF_CMD_CS_DISABLE", "OCP_IF_CMD_CS_CONTROLLER_IF", "OCP_IF_CMD_CS_HARDWARE_IF", "OCP_IF_CMD_CS_GET_NUMBER_CONTROLLERS", "OCP_IF_CMD_CS_GET_CONTROLLERS_NAMES", "OCP_IF_CMD_PLATFORM_ID", "OCP_IF_CMD_PLATFORM_IF", "OCP_IF_CMD_OPIL_UPDATE_MEASUREMENTS", "OCP_IF_CMD_OPIL_UPDATE_SIM_DATA", "OCP_IF_CMD_OPIL_RUN_CONTROL", "OCP_IF_CMD_OPIL_INITIALIZE_CONTROL", "OCP_IF_CMD_OPIL_GET_CONTROL", "OCP_IF_CMD_OPIL_GET_CONTROLLER_DATA", "OCP_IF_CMD_END"] ("CMD")
            # "pending to define"
            n156 = property on="# Control" class="CmbBox"() -> ("Value"=w433:string, "Strings[]"=w434:string[])  [unwired: 2 in, 2 out]
            n157 = Search 1D Array(1D array=w434, element=w433) -> (index of element=w430:i32)  [unwired: 1 in]
            n158 = Less Than 0?(x=w430) -> (x < 0?=w432:bool)
            n159 = Select(t=0, s=w432, f=w430) -> (s? t:f=w429:i32)
            n160 = To Long Integer(number=w429) -> (32bit integer=w428:i32)
            n161 = Bundle By Name(cluster=w441, "CS_ID"=w428) -> (w438:T6)
            n162 = call "TCP Client_33.vi"("CMD"=w440, "Input Cluster"=w438, "error in (no error)"=w436, "Comunication Cluster"=w435) -> ("Output cluster"=w442:T11, "error out"=w437:errorcluster)  [unwired: 4 in, 1 out]
            n163 = Unbundle By Name(w442) -> ("CS STATUS"=→"Current CS status":i32)
          }
        }
        n164 = call <vilib>:"Simple Error Handler.vi"("error in (no error)"=w412) -> ()  [unwired: 4 in, 5 out]
      }
      event "CS enable": Value Change {
        n165 = event-data() -> ()  [unwired: 1 in, 6 out]
        n166 = Unbundle By Name(w444) -> ("Port"=w449:i32, "hostname"=w451:string, "timeout ms"=w450:i32)
        n167 = Bundle By Name(cluster=w454, "timeout ms"=w450, "remote port"=w449, "Address"=w451) -> (w452:T7)
        n168 = flat-sequence {
          tunnel: w453 -> [w463]
          tunnel: w452 -> [w461]
          tunnel: ["CS enable"] -> w448
          tunnel: [w461] -> w447
          tunnel: [w460] -> w446
          tunnel: [w455] -> w443
          tunnel: w448 -> [w477]
          tunnel: w447 -> [w475]
          tunnel: w446 -> [w476]
          tunnel: w444 -> [w473]
          tunnel: [w472] -> w445
          tunnel: w443 -> [w471]
          frame #0 {
            n169 = property on="# Control" class="CmbBox"() -> ("Value"=w464:string, "Strings[]"=w465:string[])  [unwired: 2 in, 2 out]
            n170 = Search 1D Array(1D array=w465, element=w464) -> (index of element=w458:i32)  [unwired: 1 in]
            n171 = Less Than 0?(x=w458) -> (x < 0?=w459:bool)
            n172 = Select(t=0, s=w459, f=w458) -> (s? t:f=w456:i32)
            n173 = To Long Integer(number=w456) -> (32bit integer=w455:i32)
            n174 = Bundle By Name(cluster=w463, "CS_ID"=w455) -> (w460:T6)
          }
          frame #1 {
            n175 = case shown="False" w477 {
              selector: w477 -> [w479 w489]
              tunnel: w475 -> [w483 w494]
              tunnel: w476 -> [w480 w491]
              tunnel: [w481 w492] -> w474
              tunnel: [w479 w488] -> w469
              tunnel: w471 -> [_ w487]
              tunnel: [0 w487] -> w470
              frame False {
                w482 = 11 items=["OCP_IF_CMD_TRACE_READ", "OCP_IF_CMD_TRACE_RESET", "OCP_IF_CMD_TRACE_GET_SIZE", "OCP_IF_CMD_TRACE_SET_SIZE", "OCP_IF_CMD_TRACE_GET_NUMBER_SIGNALS", "OCP_IF_CMD_TRACE_GET_SIGNALS_NAMES", "OCP_IF_CMD_TRACE_GET_NUMBER_TRACES", "OCP_IF_CMD_TRACE_GET_TRACES_NAMES", "OCP_IF_CMD_TRACE_GET_ADDRESS", "OCP_IF_CMD_CS_STATUS", "OCP_IF_CMD_CS_ENABLE", "OCP_IF_CMD_CS_DISABLE", "OCP_IF_CMD_CS_CONTROLLER_IF", "OCP_IF_CMD_CS_HARDWARE_IF", "OCP_IF_CMD_CS_GET_NUMBER_CONTROLLERS", "OCP_IF_CMD_CS_GET_CONTROLLERS_NAMES", "OCP_IF_CMD_PLATFORM_ID", "OCP_IF_CMD_PLATFORM_IF", "OCP_IF_CMD_OPIL_UPDATE_MEASUREMENTS", "OCP_IF_CMD_OPIL_UPDATE_SIM_DATA", "OCP_IF_CMD_OPIL_RUN_CONTROL", "OCP_IF_CMD_OPIL_INITIALIZE_CONTROL", "OCP_IF_CMD_OPIL_GET_CONTROL", "OCP_IF_CMD_OPIL_GET_CONTROLLER_DATA", "OCP_IF_CMD_END"] ("CMD")
                n176 = call "TCP Client_33.vi"("CMD"=w482, "Input Cluster"=w480, "Comunication Cluster"=w483) -> ("error out"=w481:errorcluster)  [unwired: 5 in, 2 out]
              }
              frame True {
                w493 = 10 items=["OCP_IF_CMD_TRACE_READ", "OCP_IF_CMD_TRACE_RESET", "OCP_IF_CMD_TRACE_GET_SIZE", "OCP_IF_CMD_TRACE_SET_SIZE", "OCP_IF_CMD_TRACE_GET_NUMBER_SIGNALS", "OCP_IF_CMD_TRACE_GET_SIGNALS_NAMES", "OCP_IF_CMD_TRACE_GET_NUMBER_TRACES", "OCP_IF_CMD_TRACE_GET_TRACES_NAMES", "OCP_IF_CMD_TRACE_GET_ADDRESS", "OCP_IF_CMD_CS_STATUS", "OCP_IF_CMD_CS_ENABLE", "OCP_IF_CMD_CS_DISABLE", "OCP_IF_CMD_CS_CONTROLLER_IF", "OCP_IF_CMD_CS_HARDWARE_IF", "OCP_IF_CMD_CS_GET_NUMBER_CONTROLLERS", "OCP_IF_CMD_CS_GET_CONTROLLERS_NAMES", "OCP_IF_CMD_PLATFORM_ID", "OCP_IF_CMD_PLATFORM_IF", "OCP_IF_CMD_OPIL_UPDATE_MEASUREMENTS", "OCP_IF_CMD_OPIL_UPDATE_SIM_DATA", "OCP_IF_CMD_OPIL_RUN_CONTROL", "OCP_IF_CMD_OPIL_INITIALIZE_CONTROL", "OCP_IF_CMD_OPIL_GET_CONTROL", "OCP_IF_CMD_OPIL_GET_CONTROLLER_DATA", "OCP_IF_CMD_END"] ("CMD")
                n177 = call "TCP Client_33.vi"("CMD"=w493, "Input Cluster"=w491, "Comunication Cluster"=w494) -> ("Output cluster"=w490:T11, "error out"=w492:errorcluster)  [unwired: 5 in, 1 out]
                n178 = Unbundle By Name(w490) -> ("SIZE"=w486:i32)
                n179 = Not A Number/Path/Refnum?(number/path/refnum=w486) -> (NaN/Path/Refnum?=w485:bool)
                n180 = Not(x=w485) -> (.not. x?=w484:bool)
                n181 = And(x=w484, y=w489) -> (x .and. y?=w488:bool)
              }
            }
            n182 = Bundle By Name(cluster=w473, "CS enable?"=w469, "CS ID"=w470) -> (w472:T3)
            n183 = Select(t=cluster{u32, u32}[] [{3381759, 3381759}] ("Colors [4]"), s=w469, f=cluster{u32, u32}[] [{11776947, 11776947}] ("Colors [4]")) -> (s? t:f=w468:cluster{u32, u32}[])
            n184 = property on="CS enable" class="Bool (strict)"("Colors [4]"=w468) -> ()  [unwired: 2 in, 2 out]
            n185 = call <vilib>:"Simple Error Handler.vi"("error in (no error)"=w474) -> ()  [unwired: 4 in, 5 out]
          }
        }
      }
      event "Save CTRL parameters": Value Change {
        n186 = event-data() -> ()  [unwired: 1 in, 6 out]
        n187 = Unbundle By Name(w510) -> ("Port"=w506:i32, "hostname"=w505:string, "timeout ms"=w504:i32, "CS enable?"=w496:bool, "CS ID"=w497:i32)
        n188 = Bundle By Name(cluster=w507, "timeout ms"=w504, "remote port"=w506, "Address"=w505) -> (w503:T7)
        n189 = Bundle By Name(cluster=w502, "CS_ID"=w497) -> (w498:T5)
        n190 = And(x="Save CTRL parameters", y=w496) -> (x .and. y?=w508:bool)
        n191 = case shown="True" w508 {
          selector: w508 -> [w515 w533]
          tunnel: w503 -> [w532 _]
          tunnel: w511 -> [w530 w534]
          tunnel: w498 -> [w531 _]
          tunnel: [w529 w534] -> w501
          tunnel: "CS_IF_Params" -> [w528 _]
          tunnel: T10."little-endian" ("byte order (0:big-endian, network order)") -> [w527 _]
          tunnel: [w514 w533] -> w495
          frame True {
            w526 = 12 items=["OCP_IF_CMD_TRACE_READ", "OCP_IF_CMD_TRACE_RESET", "OCP_IF_CMD_TRACE_GET_SIZE", "OCP_IF_CMD_TRACE_SET_SIZE", "OCP_IF_CMD_TRACE_GET_NUMBER_SIGNALS", "OCP_IF_CMD_TRACE_GET_SIGNALS_NAMES", "OCP_IF_CMD_TRACE_GET_NUMBER_TRACES", "OCP_IF_CMD_TRACE_GET_TRACES_NAMES", "OCP_IF_CMD_TRACE_GET_ADDRESS", "OCP_IF_CMD_CS_STATUS", "OCP_IF_CMD_CS_ENABLE", "OCP_IF_CMD_CS_DISABLE", "OCP_IF_CMD_CS_CONTROLLER_IF", "OCP_IF_CMD_CS_HARDWARE_IF", "OCP_IF_CMD_CS_GET_NUMBER_CONTROLLERS", "OCP_IF_CMD_CS_GET_CONTROLLERS_NAMES", "OCP_IF_CMD_PLATFORM_ID", "OCP_IF_CMD_PLATFORM_IF", "OCP_IF_CMD_OPIL_UPDATE_MEASUREMENTS", "OCP_IF_CMD_OPIL_UPDATE_SIM_DATA", "OCP_IF_CMD_OPIL_RUN_CONTROL", "OCP_IF_CMD_OPIL_INITIALIZE_CONTROL", "OCP_IF_CMD_OPIL_GET_CONTROL", "OCP_IF_CMD_OPIL_GET_CONTROLLER_DATA", "OCP_IF_CMD_END"] ("CMD")
            n192 = Unbundle By Name(w528) -> ("SET_PARAMETERS"=w523:i32, "CTLR"=w522:i32, "CS_Duty"=w521:sgl)
            n193 = Wait (ms)(milliseconds to wait=u32 200) -> ()  [unwired: 1 out]
            n194 = Flatten To String(anything=w523, prepend array or string size? (T)=w515, byte order (0:big-endian, network order)=w527, error in (no error)=w530) -> (data string=w520:string, error out=w525:errorcluster)  [unwired: 1 out]
            n195 = Flatten To String(anything=w522, prepend array or string size? (T)=w515, byte order (0:big-endian, network order)=w527, error in (no error)=w525) -> (data string=w519:string, error out=w524:errorcluster)  [unwired: 1 out]
            n196 = Flatten To String(anything=w521, prepend array or string size? (T)=w515, byte order (0:big-endian, network order)=w527, error in (no error)=w524) -> (data string=w518:string, error out=w513:errorcluster)  [unwired: 1 out]
            n197 = Concatenate Strings(w520, w519, w518) -> (w516:string)
            n198 = Not(x=w515) -> (.not. x?=w514:bool)
            n199 = Bundle By Name(cluster=w531, "DATA PARAM"=w516) -> (w517:T5)
            n200 = call "TCP Client_34.vi"("CMD"=w526, "Input Cluster"=w517, "error in (no error)"=w513, "Comunication Cluster"=w532) -> ("error out"=w529:errorcluster)  [unwired: 4 in, 2 out]
          }
          frame False {
          }
        }
        n201 = call <vilib>:"Simple Error Handler.vi"("error in (no error)"=w501) -> ()  [unwired: 4 in, 5 out]
        n202 = local write "Save CTRL parameters"(w495) -> ()
      }
      event "CTRL enable": Value Change {
        w540 = TRUE
        w547 = 12 items=["OCP_IF_CMD_TRACE_READ", "OCP_IF_CMD_TRACE_RESET", "OCP_IF_CMD_TRACE_GET_SIZE", "OCP_IF_CMD_TRACE_SET_SIZE", "OCP_IF_CMD_TRACE_GET_NUMBER_SIGNALS", "OCP_IF_CMD_TRACE_GET_SIGNALS_NAMES", "OCP_IF_CMD_TRACE_GET_NUMBER_TRACES", "OCP_IF_CMD_TRACE_GET_TRACES_NAMES", "OCP_IF_CMD_TRACE_GET_ADDRESS", "OCP_IF_CMD_CS_STATUS", "OCP_IF_CMD_CS_ENABLE", "OCP_IF_CMD_CS_DISABLE", "OCP_IF_CMD_CS_CONTROLLER_IF", "OCP_IF_CMD_CS_HARDWARE_IF", "OCP_IF_CMD_CS_GET_NUMBER_CONTROLLERS", "OCP_IF_CMD_CS_GET_CONTROLLERS_NAMES", "OCP_IF_CMD_PLATFORM_ID", "OCP_IF_CMD_PLATFORM_IF", "OCP_IF_CMD_OPIL_UPDATE_MEASUREMENTS", "OCP_IF_CMD_OPIL_UPDATE_SIM_DATA", "OCP_IF_CMD_OPIL_RUN_CONTROL", "OCP_IF_CMD_OPIL_INITIALIZE_CONTROL", "OCP_IF_CMD_OPIL_GET_CONTROL", "OCP_IF_CMD_OPIL_GET_CONTROLLER_DATA", "OCP_IF_CMD_END"] ("CMD")
        w553 = T10."little-endian" ("byte order (0:big-endian, network order)")
        n203 = event-data() -> ()  [unwired: 1 in, 6 out]
        n204 = Unbundle By Name(w561) -> ("Port"=w559:i32, "hostname"=w558:string, "timeout ms"=w557:i32, "CS enable?"=w551:bool, "CS ID"=w552:i32)
        n205 = Bundle By Name(cluster=w560, "timeout ms"=w557, "remote port"=w559, "Address"=w558) -> (w556:T7)
        n206 = Bundle By Name(cluster=w555, "CS_ID"=w552) -> (w549:T5)
        n207 = local read "CS_IF_Params"() -> (w548:T2)
        n208 = And(x="CTRL enable", y=w551) -> (x .and. y?=w538:bool)
        n209 = Unbundle By Name(w548) -> ("CTRL_IF_SET"=w539:i32)
        n210 = Flatten To String(anything=w539, prepend array or string size? (T)=w540, byte order (0:big-endian, network order)=w553, error in (no error)=w562) -> (data string=w545:string, error out=w546:errorcluster)  [unwired: 1 out]
        n211 = Select(t=2 ("CTRL_IF_SET"), s=w538, f=0 ("CTRL_IF_SET")) -> (s? t:f=w536:i32)
        n212 = Flatten To String(anything=w536, prepend array or string size? (T)=w540, byte order (0:big-endian, network order)=w553, error in (no error)=w546) -> (data string=w544:string, error out=w543:errorcluster)  [unwired: 1 out]
        n213 = Concatenate Strings(w545, w544) -> (w542:string)
        n214 = Bundle By Name(cluster=w549, "DATA PARAM"=w542) -> (w541:T5)
        n215 = call "TCP Client_34.vi"("CMD"=w547, "Input Cluster"=w541, "error in (no error)"=w543, "Comunication Cluster"=w556) -> ("error out"=w554:errorcluster)  [unwired: 4 in, 2 out]
        n216 = call <vilib>:"Simple Error Handler.vi"("error in (no error)"=w554) -> ()  [unwired: 4 in, 5 out]
      }
    }
    n217 = property on="Multicolumn Listbox" class="MCListbox (strict)"() -> ("ItemNames"=w51:string[][])  [unwired: 2 in, 2 out]
    n218 = Index Array(array=w48, index=0) -> (element=w47:refnum<queue>)
    n219 = case shown="True" "Send message" {
      tunnel: w51 -> [_ w68]
      tunnel: w50 -> [_ w70]
      tunnel: w47 -> [_ w69]
      frame False {
      }
      frame True {
        n220 = Array Size(array=w68) -> (size(s)=w66:i32[])
        n221 = case shown="Default" "Process 2" {
          selector: "Process 2" -> [w88 _]
          tunnel: w68 -> [w90 _]
          tunnel: w70 -> [w78 _]
          tunnel: w69 -> [w79 _]
          frame Default {
            w74 = FALSE ("create if not found? (T)")
            n222 = Get Queue Status(queue=w79, error in (no error)=w78) -> (error out=w76:errorcluster)  [unwired: 1 in, 7 out]
            n223 = Index Array(array=w90, index (row)=w88, index (col)=0 ("disabled index (col)")) -> (element=w72:string)
            n224 = local write "Send message"(w74) -> ()
            n225 = Obtain Queue(name (unnamed)=w72, element data type="", create if not found? (T)=w74, error in (no error)=w76) -> (queue out=w77:refnum<queue>, error out=w75:errorcluster)  [unwired: 1 in, 1 out]
            n226 = Concatenate Strings("message::", "msj") -> (w83:string)
            n227 = Get Queue Status(queue=w77, error in (no error)=w75) -> (queue out=w87:refnum<queue>, error out=w86:errorcluster)  [unwired: 1 in, 6 out]
            n228 = Enqueue Element(queue=w87, element=w83, error in (no error)=w86) -> (queue out=w82:refnum<queue>, error out=w81:errorcluster)  [unwired: 1 in, 1 out]
            n229 = Release Queue(queue=w82, error in (no error)=w81) -> (error out=w80:errorcluster)  [unwired: 1 in, 2 out]
            n230 = call <vilib>:"Simple Error Handler.vi"("error in (no error)"=w80) -> ()  [unwired: 4 in, 5 out]
          }
          frame ..-1 {
          }
        }
        n231 = Index Array(array=w66, index=0) -> (element=w65:i32)
        n232 = property on="Process 2" class="DigNum (strict)"("Maximum"=w65) -> ()  [unwired: 2 in, 2 out]
      }
    }
    n233 = Dequeue Element(queue=w62, timeout in ms (-1)=100, error in (no error)=w58) -> (queue out=w59:refnum<queue>, element=w61:string, timed out?=w60:bool, error out=w53:errorcluster)
    n234 = case shown="False" w60 {
      tunnel: w61 -> [w93 _]
      frame False {
        n235 = Match Pattern(string=w93, regular expression="::") -> (before substring=w92:string, after substring=w91:string)  [unwired: 1 in, 2 out]
        n236 = case shown="\"process started\"" w92 {
          tunnel: w91 -> [_ w103 w108]
          frame "False", Default {
            # "unhandled received commands."
            n237 = call <vilib>:"Error Cluster From Error Code.vi"("error message (\"\")"="Invalid command received from process VI" ("error message (\"\")"), "error code (0)"=1) -> ("error out"=w95:errorcluster)  [unwired: 7 in]
            n238 = call <vilib>:"Simple Error Handler.vi"("error in (no error)"=w95) -> ()  [unwired: 4 in, 5 out]
          }
          frame "process stopped" {
            n239 = property on="Multicolumn Listbox" class="MCListbox (strict)"() -> ("ItemNames"=w99:string[][])  [unwired: 2 in, 2 out]
            n240 = Index Array(array=w99, index (col)=0 ("disabled index (col)")) -> (element=w100:string[])  [unwired: 1 in]
            n241 = Search 1D Array(1D array=w100, element=w103) -> (index of element=w101:i32)  [unwired: 1 in]
            n242 = Delete From Array(array=w99, index (row)=w101) -> (array with subset deleted=w98:string[][])  [unwired: 2 in, 1 out]
            n243 = property on="Multicolumn Listbox" class="MCListbox (strict)"("ItemNames"=w98) -> ()  [unwired: 2 in, 2 out]
          }
          frame "process started" {
            n244 = Build Array(w108, "" ("element")) -> (w106:string[])
            n245 = property on="Multicolumn Listbox" class="MCListbox (strict)"() -> ("ItemNames"=w105:string[][])  [unwired: 2 in, 2 out]
            n246 = Build Array (concatenate)(w105, w106) -> (w104:string[][])
            n247 = property on="Multicolumn Listbox" class="MCListbox (strict)"("ItemNames"=w104) -> ()  [unwired: 2 in, 2 out]
          }
        }
      }
      frame True {
      }
    }
  }
  n248 = invoke on="Size bytes X #Traces" class="DigNum (strict)" method="Reinit To Default"(error in=w14) -> (error out=w13:errorcluster)  [unwired: 2 in, 2 out]
  n249 = shared-variable ".\\Variable 1.lvlib\\Close_all_wplots"(FALSE ("Close_all_wplots"), error in=w13) -> (error out=w19:errorcluster)
  n250 = invoke on="Multicolumn Listbox" class="MCListbox (strict)" method="Reinit To Default"(error in=w19) -> (error out=w24:errorcluster)  [unwired: 2 in, 2 out]
  n251 = property on="Multicolumn Listbox" class="MCListbox (strict)"(error in=w24, "ItemNames"=string[][] [] ("Item Names")) -> (error out=w12:errorcluster)  [unwired: 1 in, 1 out]
  n252 = property on="New plot" class="Bool (strict)"(error in=w12, "Value"=FALSE ("New plot"), "Visible"=TRUE, "DisabledEnum"=T4."Enabled" ("Disabled")) -> (error out=w11:errorcluster)  [unwired: 1 in, 1 out]
  n253 = property on="Close All plots" class="Bool (strict)"(error in=w11, "Value"=FALSE ("Cancel Button")) -> (error out=w2:errorcluster)  [unwired: 1 in, 1 out]
  n254 = shared-variable ".\\Variable 1.lvlib\\Signals_value_Array"(dbl[] [] ("Signals_value_Array"), error in=w2) -> (error out=w8:errorcluster)
  n255 = property on="CS enable" class="Bool (strict)"(error in=w8, "Colors [4]"=cluster{u32, u32}[] [{11776947, 11776947}]) -> (error out=w6:errorcluster)  [unwired: 1 in, 1 out]
  n256 = property on="Refresh \ntime (ms)" class="DigNum (strict)"(error in=w6, "Value"=500 ("Refresh \ntime (ms)")) -> (error out=w5:errorcluster)  [unwired: 1 in, 1 out]
  n257 = call <vilib>:"Simple Error Handler.vi"("error in (no error)"=w5) -> ()  [unwired: 4 in, 5 out]
  n258 = Flush Queue(queue=w26) -> ()  [unwired: 1 in, 3 out]
  n259 = for {
    tunnel: w40 -> [w564] mode=indexing
    n260 = Release Queue(queue=w564, force destroy? (F)=FALSE) -> ()  [unwired: 1 in, 3 out]
  }
  n261 = Release Queue(queue=w26, error in (no error)=w35) -> (error out=w33:errorcluster)  [unwired: 1 in, 2 out]
  n262 = property on="Multicolumn Listbox" class="MCListbox (strict)"(error in=w33) -> (error out=w29:errorcluster, "ItemNames"=w32:string[][])  [unwired: 1 in, 1 out]
  n263 = Index Array(array=w32, index (col)=0 ("disabled index (col)")) -> (element=w30:string[])  [unwired: 1 in]
  n264 = for {
    tunnel: w30 -> [w574] mode=indexing
    shift-right: [w571] -> w28
    shift-left: w29 -> [w573]
    n265 = Obtain Queue(name (unnamed)=w574, element data type="", error in (no error)=w573) -> (queue out=w566:refnum<queue>, error out=w568:errorcluster)  [unwired: 2 in, 1 out]
    n266 = Enqueue Element(queue=w566, element="exit::", error in (no error)=w568) -> (queue out=w565:refnum<queue>, error out=w567:errorcluster)  [unwired: 1 in, 1 out]
    n267 = Release Queue(queue=w565, force destroy? (F)=FALSE, error in (no error)=w567) -> (error out=w571:errorcluster)  [unwired: 2 out]
  }
  n268 = call <vilib>:"Simple Error Handler.vi"("error in (no error)"=w28) -> ("error out"=w27:errorcluster)  [unwired: 4 in, 4 out]
  n269 = flat-sequence {
    tunnel: w27 -> [_]
    frame #0 {
      n270 = property class="App"() -> ("App.Kind"=w578:T12)  [unwired: 2 in, 2 out]
      n271 = Equal?(x=w578, y=T12."Run Time System" ("Application:Kind")) -> (x = y?=→"Close":bool)
      n272 = Quit LabVIEW(quit? (T)=TRUE) -> ()
    }
  }
